vi "GDSLvClass_SaveEverythingInClass.vi"(0 "ClassRefIn":refnum<vi>, 1 "ForceResaving(False)":bool, 5 "error in":errorcluster) -> (14 "ClassRefOut":refnum<vi>, 19 "error out":errorcluster)   [LabVIEW 2020]
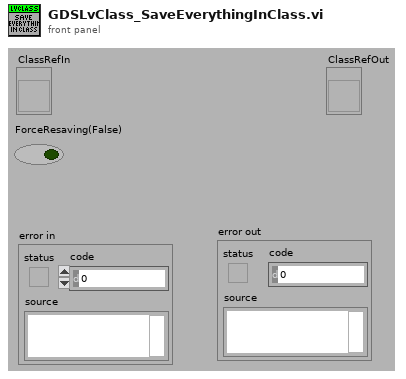
[diagram p1: front panel]
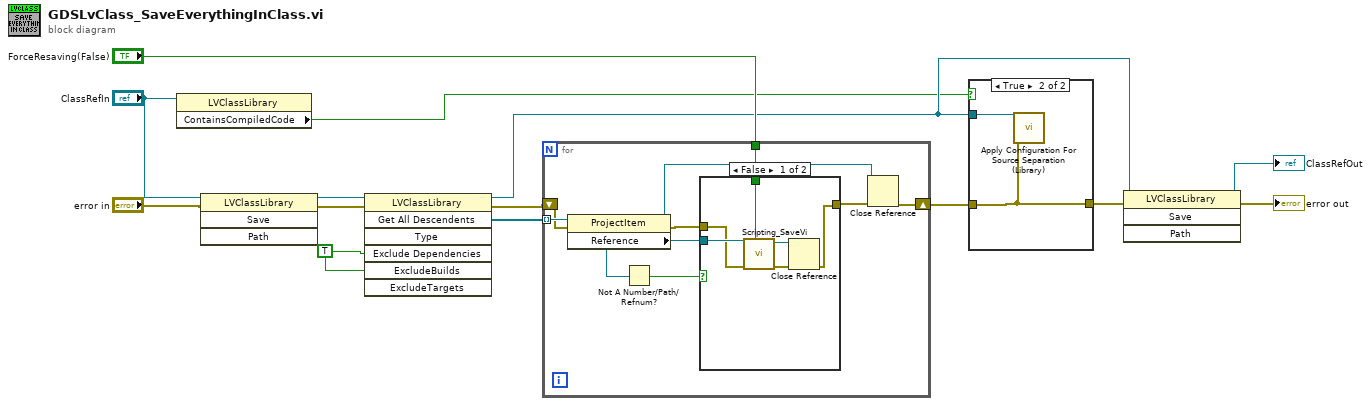
[diagram p0: block diagram]
diagram:
  w6 = TRUE ("ExcludeDependencies")
  n1 = property class="LVClassLibrary"(reference="ClassRefIn") -> ("ContainsCompiledCode"=w3:bool)  [unwired: 1 in, 2 out]
  n2 = invoke class="LVClassLibrary" method="Save"(reference="ClassRefIn", error in="error in") -> (reference out=w13:refnum<vi>, error out=w12:errorcluster)  [unwired: 2 in, 2 out]
  n3 = invoke class="LVClassLibrary" method="Get All Descendents"(reference=w13, error in=w12, "Exclude Dependencies"=w6, "ExcludeBuilds"=w6) -> (reference out=w5:refnum<vi>, error out=w10:errorcluster, "All Descendents"=w11:refnum<vi>[])  [unwired: 3 in, 4 out]
  n4 = for {
    tunnel: w11 -> [w23] mode=indexing
    shift-right: [w16] -> w2
    shift-left: w10 -> [w19]
    tunnel: "ForceResaving(False)" -> [w18]
    n5 = property class="ProjectItem"(reference=w23, error in=w19) -> (reference out=w15:refnum<vi>, error out=w20:errorcluster, "Reference"=w21:refnum<vi>)
    n6 = Not A Number/Path/Refnum?(number/path/refnum=w21) -> (NaN/Path/Refnum?=w22:bool)
    n7 = case shown="False" w22 {
      tunnel: w21 -> [w29 _]
      tunnel: w20 -> [w28 w30]
      tunnel: [w25 w30] -> w17
      tunnel: w18 -> [w24 _]
      frame False {
        n8 = call <resource>:"Scripting_SaveVi.vi"("ForceResaving(False)"=w24, "error in (no error)"=w28, "VIRefToSaveIn"=w29) -> ("error out"=w27:errorcluster, "VIRefToSaveOut"=w26:refnum<vi>)  [unwired: 7 in]
        n9 = Close Reference(reference=w26, error in (no error)=w27) -> (error out=w25:errorcluster)
      }
      frame True {
      }
    }
    n10 = Close Reference(reference=w15, error in (no error)=w17) -> (error out=w16:errorcluster)
  }
  n11 = case shown="True" w3 {
    tunnel: w5 -> [_ w33]
    tunnel: w2 -> [w31 w32]
    tunnel: [w31 w32] -> w1
    frame False {
    }
    frame True {
      n12 = call <vilib>:"Apply Configuration For Source Separation (Library).vi"("error in (no error)"=w32, "Library in"=w33) -> ()  [unwired: 8 in, 2 out]
    }
  }
  n13 = invoke class="LVClassLibrary" method="Save"(reference=w5, error in=w1) -> (reference out=→"ClassRefOut":refnum<vi>, error out=→"error out":errorcluster)  [unwired: 2 in, 2 out]
